vi "Delete Table turnos.vi"(8 "error in (no error)":errorcluster, 11 "Contabilidad in":refnum<class "Contabilidad.lvclass">) -> (0 "error out":errorcluster, 3 "Contabilidad out":refnum<class "Contabilidad.lvclass">)   [LabVIEW 2020, in "Contabilidad.lvlib" / "Contabilidad.lvclass"]
uses:
  Contabilidad.lvclass
  <vilib>/drjdpowell/SQLite Library/SQL Connection/Open (path).vi
  <vilib>/drjdpowell/SQLite Library/SQL Connection/Open (string).vi
  <vilib>/AdvancedString/Path To Command Line String.vi
  <vilib>/drjdpowell/SQLite Library/SQL Connection/Execute SQL.vi
  <vilib>/drjdpowell/SQLite Library/SQL Connection/Connection.lvclass
  <vilib>/drjdpowell/SQLite Library/SQLite.lvlib
panel:
  out "Servicio Estatus":string[][](array[string])
  in  "error in (no error) 2":errorcluster
  out "error out 2":errorcluster
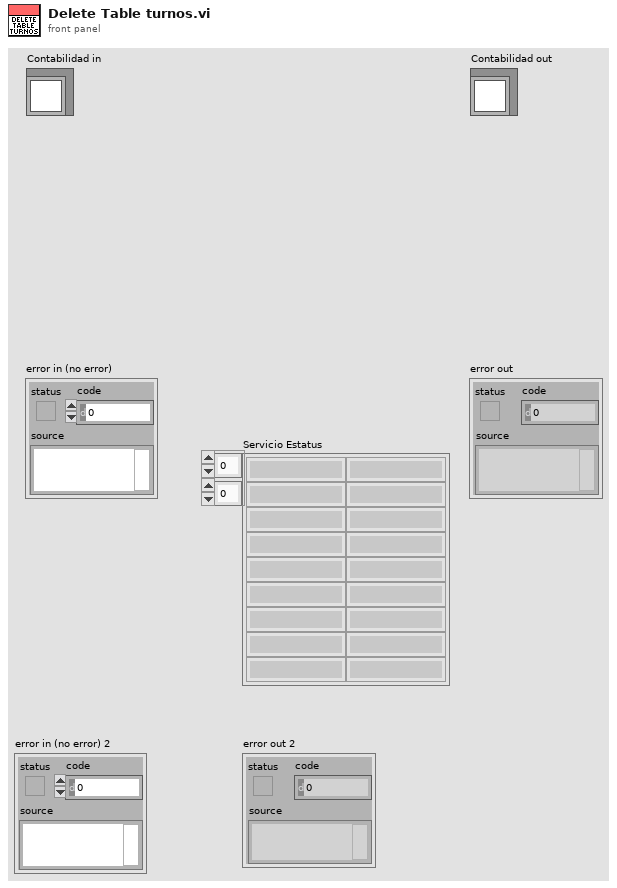
[diagram p1: front panel]
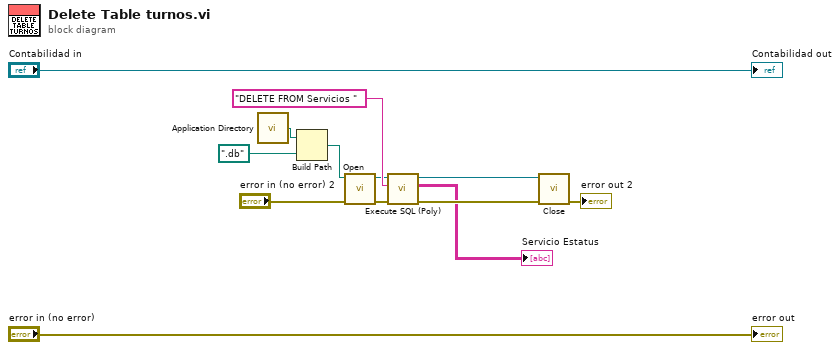
[diagram p0: block diagram]
diagram:
  n1 = call <vilib>:"Application Directory.vi"() -> ("Application Directory"=w8:path)
  n2 = Build Path(base path=w8, name or relative path=path ".db") -> (appended path=w6:path)
  n3 = call-poly <vilib>:"Open.vi"("error in (no error)"="error in (no error) 2", "db file"=w6) -> ("error out"=w10:errorcluster, "SQLite Connection"=w5:refnum<class "Connection.lvclass">)  [unwired: 8 in]
  n4 = call-poly <vilib>:"Execute SQL (Poly).vi"("error in (no error)"=w10, "SQL"="DELETE FROM Servicios ", "SQLite Connection in"=w5) -> ("error out"=w11:errorcluster, "Result Set"=→"Servicio Estatus":string[][], "SQLite Connection"=w4:refnum<class "Connection.lvclass">)  [unwired: 5 in, 1 out]
  n5 = call-dynamic "Close.vi"("error in (no error)"=w11, "SQLite Connection in"=w4) -> ("error out"=→"error out 2":errorcluster)  [unwired: 9 in]
  "error out" <- "error in (no error)"
  "Contabilidad out" <- "Contabilidad in"
